vi "Polar Plot - Initialize Polar.vi"(6 "polar attributes":T2 {"minimum" format="%0.2f"; "maximum" format="%0.2f"}, 7 "[user-specified font]":T4, 11 "rect":T5={"left"=0, "top"=0, "right"=324, "bottom"=234}) -> (2 "grid measurements":T1 {"end angle" format="%0.2f"; "start angle" format="%0.2f"; "scale factors"."b" format="%0.2f"; "scale factors"."a" format="%0.2f"}, 3 "scale specs":cluster{"coordinate":i16, "label":string}[](array[cluster])=[{"coordinate"=7, "label"="1"}, {"coordinate"=23, "label"="2"}])   [LabVIEW 2020]
panel:
  in  "look up table":cluster{dbl, dbl}[](array[cluster])=[{0.0, 90.0}, {270.0, 360.0}, {180.0, 270.0}, {90.0, 180.0}, {0.0, 180.0}, {180.0, 360.0}, {270.0, 450.0}, {90.0, 270.0}, {0.0, 360.0}] {"?" format="%0.2f"; "?" format="%0.2f"}
  in  "desired font(Application)":T3(ring)=enum."Application Font"
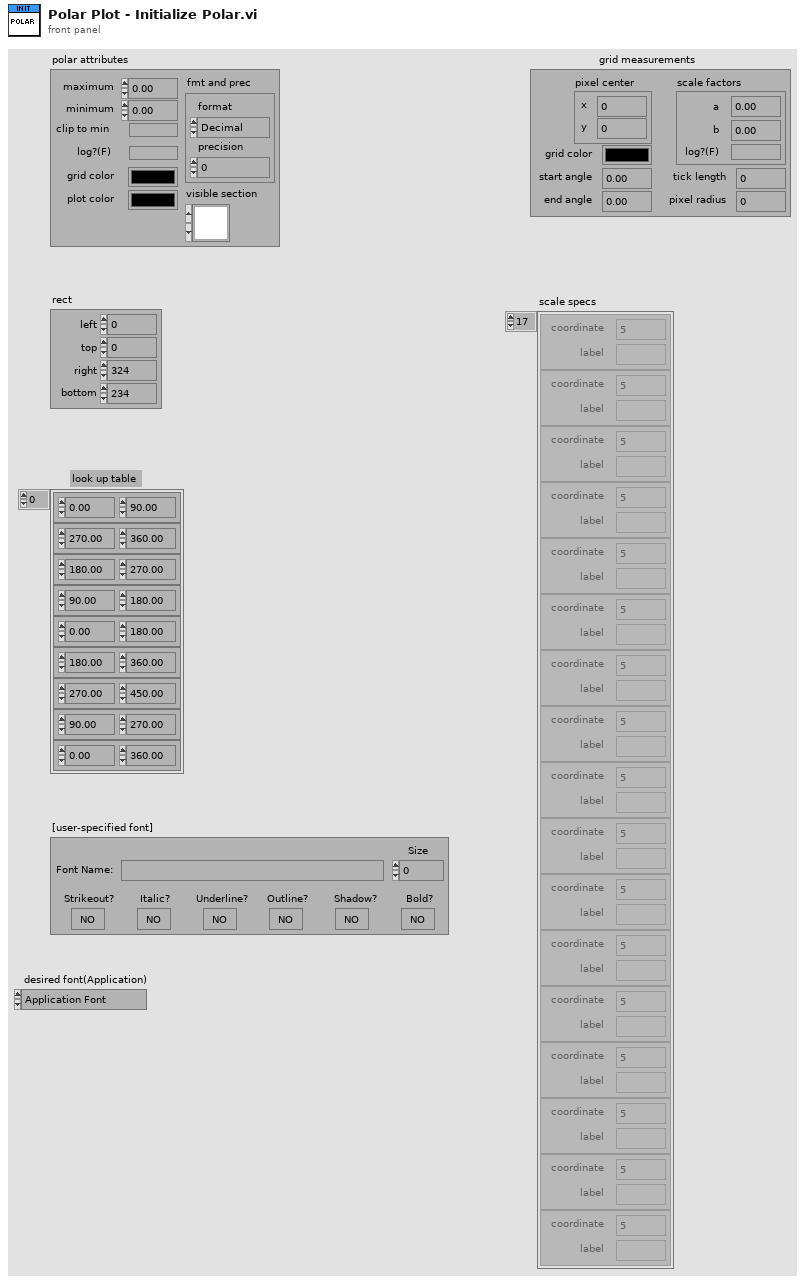
[diagram p1: front panel]
types:
  T1 = cluster{"pixel center":cluster{"x":i16, "y":i16}, "scale factors":cluster{"a":dbl, "b":dbl, "log?(F)":bool}, "grid color":u32, "start angle":dbl, "end angle":dbl, "tick length":i16, "pixel radius":i32}
  T2 = cluster{"maximum":dbl, "minimum":dbl, "clip to min":bool, "log?(F)":bool, "grid color":u32, "plot color":u32, "fmt and prec":cluster{"format":enum8{"Decimal", "Scientific", "Engineering", "Binary", "Octal", "Hex"}, "precision":u8}, "visible section":u16}
  T3 = enum16{"User-specified Font", "Application Font", "System Font", "Dialog Font"}
  T4 = cluster{"Font Name:":string, "Size":i16, "Strikeout?":bool, "Italic?":bool, "Underline?":bool, "Outline?":bool, "Shadow?":bool, "Bold?":bool}
  T5 = cluster{"left":i16, "top":i16, "right":i16, "bottom":i16}
  T6 = cluster{"Coordinate 1":i32, "maximum":dbl, "Coordinate 2":i32, "minimum":dbl, "log?(F)":bool, "fmt and prec":cluster{"format":enum8{"Decimal", "Scientific", "Engineering", "Binary", "Octal", "Hex"}, "precision":u8}}
  T7 = cluster{"format":enum8{"Decimal", "Scientific", "Engineering", "Binary", "Octal", "Hex"}, "precision":u8}
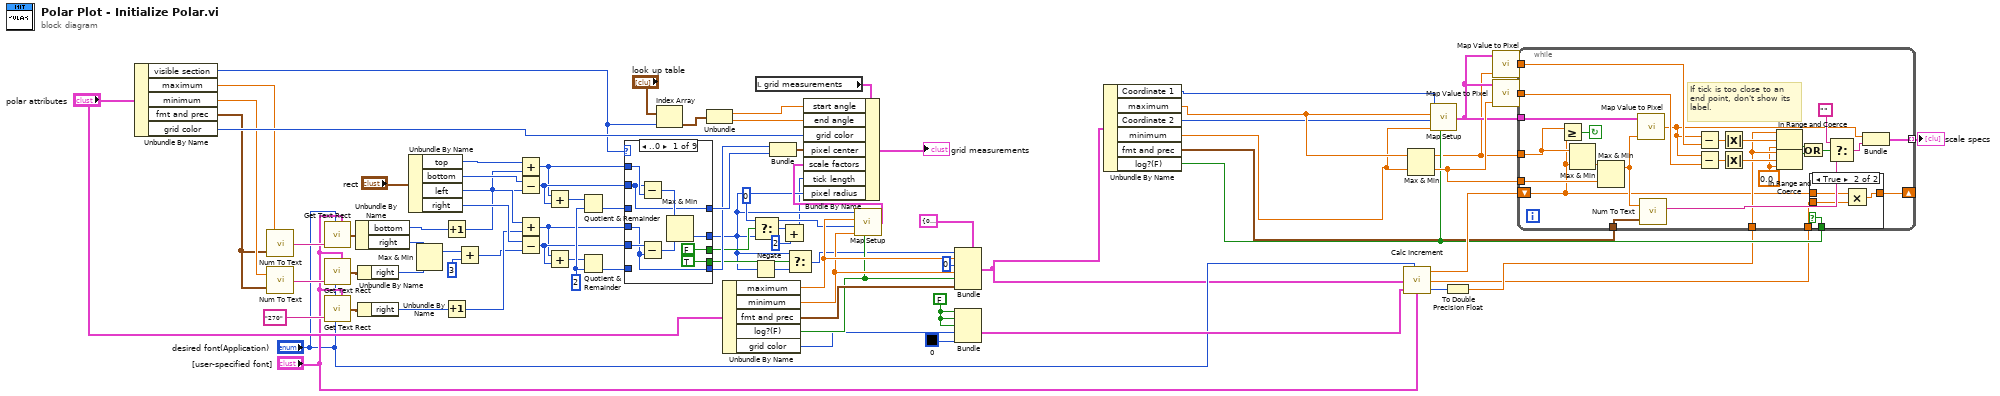
[diagram p0: block diagram]
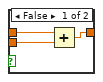
[diagram p2: hidden frame]
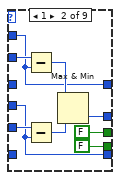
[diagram p3: hidden frame]
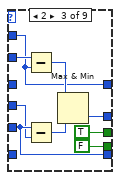
[diagram p4: hidden frame]
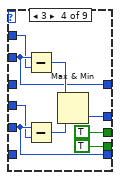
[diagram p5: hidden frame]
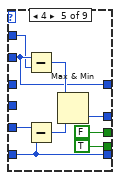
[diagram p6: hidden frame]
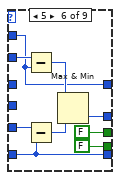
[diagram p7: hidden frame]
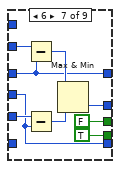
[diagram p8: hidden frame]
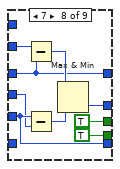
[diagram p9: hidden frame]
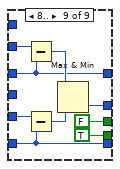
[diagram p10: hidden frame]
diagram:
  w31 = 0
  w67 = FALSE
  w78 = 2
  n1 = Unbundle By Name("polar attributes") -> ("visible section"=w25:u16, "maximum"=w54:dbl, "minimum"=w60:dbl, "fmt and prec"=w53:T7, "grid color"=w68:u32)
  n2 = call <vilib>:"Num To Text.vi"("fmt and prec"=w53, "number"=w54) -> ("numeric string"=w52:string)
  n3 = call <vilib>:"Num To Text.vi"("fmt and prec"=w53, "number"=w60) -> ("numeric string"=w75:string)
  n4 = call <vilib>:"Get Text Rect.vi"("desired font(Application)"="desired font(Application)", "text"=w52, "[user-specified font]"="[user-specified font]") -> ("rect"=w51:T5)  [unwired: 6 in]
  n5 = call <vilib>:"Get Text Rect.vi"("desired font(Application)"="desired font(Application)", "text"=w75, "[user-specified font]"="[user-specified font]") -> ("rect"=w74:T5)  [unwired: 6 in]
  n6 = call <vilib>:"Get Text Rect.vi"("desired font(Application)"="desired font(Application)", "text"="270", "[user-specified font]"="[user-specified font]") -> ("rect"=w73:T5)  [unwired: 6 in]
  n7 = Unbundle By Name(w51) -> ("bottom"=w48:i16, "right"=w50:i16)
  n8 = Unbundle By Name(w74) -> ("right"=w49:i16)
  n9 = Unbundle By Name(w73) -> ("right"=w46:i16)
  n10 = Unbundle By Name("rect") -> ("top"=w82:i16, "bottom"=w81:i16, "left"=w80:i16, "right"=w79:i16)
  n11 = Max & Min(x=w50, y=w49) -> (max(x,y)=w28:i16)  [unwired: 1 out]
  n12 = Increment(x=w48) -> (x+1=w47:i16)
  n13 = Increment(x=w46) -> (x+1=w45:i16)
  n14 = Add(x=w28, y=3) -> (x+y=w29:i32)
  n15 = Add(x=w82, y=w47) -> (x+y=w39:i16)
  n16 = Subtract(x=w81, y=w47) -> (x-y=w40:i16)
  n17 = Add(x=w80, y=w45) -> (x+y=w41:i16)
  n18 = Subtract(x=w79, y=w29) -> (x-y=w42:i32)
  n19 = Add(x=w39, y=w40) -> (x+y=w77:i16)
  n20 = Add(x=w41, y=w42) -> (x+y=w76:i32)
  n21 = Quotient & Remainder(x=w77, y=w78) -> (floor(x/y)=w38:i32)  [unwired: 1 out]
  n22 = Quotient & Remainder(x=w76, y=w78) -> (floor(x/y)=w43:i32)  [unwired: 1 out]
  n23 = case shown="..0" w25 {
    tunnel: w43 -> [_ _ _ _ w124 w131 _ _ w158]
    tunnel: w42 -> [w90 w98 w105 w115 w126 w134 w141 w150 w161]
    tunnel: w41 -> [w88 w96 w104 w113 _ _ w140 w149 _]
    tunnel: w38 -> [_ _ _ _ _ _ w142 w151 w159]
    tunnel: w40 -> [w86 w99 w108 w116 w123 w135 w144 w153 w162]
    tunnel: w39 -> [w87 w95 w106 w114 w122 w132 _ _ _]
    tunnel: [w89 w97 w107 w117 w125 w133 w143 w152 w160] -> w30
    tunnel: [w86 w95 w106 w116 w123 w132 w142 w151 w159] -> w37
    tunnel: [w88 w96 w105 w115 w124 w131 w140 w150 w158] -> w36
    tunnel: [TRUE FALSE FALSE TRUE TRUE FALSE TRUE TRUE TRUE] -> w35
    tunnel: [FALSE FALSE TRUE TRUE FALSE FALSE FALSE TRUE FALSE] -> w32
    frame ..0 {
      n24 = Subtract(x=w86, y=w87) -> (x-y=w91:i16)
      n25 = Subtract(x=w90, y=w88) -> (x-y=w92:i32)
      n26 = Max & Min(x=w91, y=w92) -> (min(x,y)=w89:i32)  [unwired: 1 out]
    }
    frame 1 {
      n27 = Subtract(x=w99, y=w95) -> (x-y=w100:i16)
      n28 = Subtract(x=w98, y=w96) -> (x-y=w101:i32)
      n29 = Max & Min(x=w100, y=w101) -> (min(x,y)=w97:i32)  [unwired: 1 out]
    }
    frame 2 {
      n30 = Subtract(x=w108, y=w106) -> (x-y=w109:i16)
      n31 = Subtract(x=w105, y=w104) -> (x-y=w110:i32)
      n32 = Max & Min(x=w109, y=w110) -> (min(x,y)=w107:i32)  [unwired: 1 out]
    }
    frame 3 {
      n33 = Subtract(x=w116, y=w114) -> (x-y=w118:i16)
      n34 = Subtract(x=w115, y=w113) -> (x-y=w119:i32)
      n35 = Max & Min(x=w118, y=w119) -> (min(x,y)=w117:i32)  [unwired: 1 out]
    }
    frame 4 {
      n36 = Subtract(x=w123, y=w122) -> (x-y=w127:i16)
      n37 = Subtract(x=w126, y=w124) -> (x-y=w128:i32)
      n38 = Max & Min(x=w127, y=w128) -> (min(x,y)=w125:i32)  [unwired: 1 out]
    }
    frame 5 {
      n39 = Subtract(x=w135, y=w132) -> (x-y=w136:i16)
      n40 = Subtract(x=w134, y=w131) -> (x-y=w137:i32)
      n41 = Max & Min(x=w136, y=w137) -> (min(x,y)=w133:i32)  [unwired: 1 out]
    }
    frame 6 {
      n42 = Subtract(x=w144, y=w142) -> (x-y=w145:i32)
      n43 = Subtract(x=w141, y=w140) -> (x-y=w146:i32)
      n44 = Max & Min(x=w145, y=w146) -> (min(x,y)=w143:i32)  [unwired: 1 out]
    }
    frame 7 {
      n45 = Subtract(x=w153, y=w151) -> (x-y=w154:i32)
      n46 = Subtract(x=w150, y=w149) -> (x-y=w155:i32)
      n47 = Max & Min(x=w154, y=w155) -> (min(x,y)=w152:i32)  [unwired: 1 out]
    }
    frame 8.. {
      n48 = Subtract(x=w162, y=w159) -> (x-y=w163:i32)
      n49 = Subtract(x=w161, y=w158) -> (x-y=w164:i32)
      n50 = Max & Min(x=w163, y=w164) -> (min(x,y)=w160:i32)  [unwired: 1 out]
    }
  }
  n51 = Index Array(array="look up table", index=w25) -> (element=w64:cluster{dbl, dbl})
  n52 = Unbundle(w64) -> (w62:dbl, w63:dbl)
  n53 = Unbundle By Name("polar attributes") -> ("maximum"=w57:dbl, "minimum"=w56:dbl, "fmt and prec"=w61:T7, "log?(F)"=w55:bool, "grid color"=w24:u32)
  n54 = Negate(x=w30) -> (-x=w33:i32)
  n55 = Select(t=w31, s=w32, f=w30) -> (s? t:f=w27:i32)
  n56 = local read "grid measurements"() -> (w69:T1)
  n57 = Bundle(w36, w37) -> (w59:cluster{i32, i32})  [unwired: 1 in]
  n58 = Add(x=w27, y=2) -> (x+y=w22:i32)
  n59 = Select(t=w30, s=w35, f=w33) -> (s? t:f=w34:i32)
  n60 = call <vilib>:"Map Setup.vi"("coordinate 1"=w30, "value 1"=w57, "coordinate 2"=w31, "value 2"=w56, "log?(F)"=w55) -> ("scale factors"=w58:cluster{"a":dbl, "b":dbl, "log?(F)":bool})
  n61 = Bundle By Name(cluster=w69, "start angle"=w62, "end angle"=w63, "grid color"=w68, "pixel center"=w59, "scale factors"=w58, "tick length"=w22, "pixel radius"=w30) -> (→"grid measurements":T1)
  n62 = Bundle(cluster=T6 {"Coordinate 1"=0, "maximum"=0.0, "Coordinate 2"=0, "minimum"=0.0, "log?(F)"=FALSE, "fmt and prec"={"format"=enum."Decimal", "precision"=0}}, "Coordinate 1"=w34, "maximum"=w57, "Coordinate 2"=0, "minimum"=w56, "log?(F)"=w55, "fmt and prec"=w61) -> (w5:T6)
  n63 = Bundle(w67, w67, w67, "grid color"=w24, u32 0) -> (w14:cluster{bool, bool, bool, "grid color":u32, u32})  [unwired: 1 in]
  n64 = Unbundle By Name(w5) -> ("Coordinate 1"=w12:i32, "maximum"=w11:dbl, "Coordinate 2"=w10:i32, "minimum"=w9:dbl, "fmt and prec"=w8:T7, "log?(F)"=w7:bool)
  n65 = call <vilib>:"Calc Increment.vi"("desired font(Application)"="desired font(Application)", "scale definition"=w5, "scale attributes"=w14, "[user-specified font]"="[user-specified font]") -> ("start"=w17:dbl, "increment"=w1:dbl, "text size"=w3:i16)  [unwired: 3 in]
  n66 = Max & Min(x=w11, y=w9) -> (max(x,y)=w4:dbl, min(x,y)=w21:dbl)
  n67 = call <vilib>:"Map Setup.vi"("coordinate 1"=w12, "value 1"=w11, "coordinate 2"=w10, "value 2"=w9, "log?(F)"=w7) -> ("scale factors"=w20:cluster{"a":dbl, "b":dbl, "log?(F)":bool})
  n68 = To Double Precision Float(number=w3) -> (double precision float=w2:dbl)
  n69 = call <vilib>:"Map Value to Pixel.vi"("x"=w4, "scale factors"=w20) -> ("pixel"=w19:dbl)  [unwired: 1 in]
  n70 = call <vilib>:"Map Value to Pixel.vi"("x"=w21, "scale factors"=w20) -> ("pixel"=w18:dbl)  [unwired: 1 in]
  n71 = while {
    tunnel: w7 -> [w165]
    tunnel: w18 -> [w175]
    tunnel: w19 -> [w183]
    tunnel: w2 -> [w174]
    tunnel: w8 -> [w186]
    tunnel: [w190] -> w16 mode=indexing
    tunnel: w1 -> [w168]
    tunnel: w20 -> [w185]
    tunnel: w21 -> [w188]
    tunnel: w4 -> [w187]
    shift-left: w17 -> [w167]
    shift-right: [w166] -> _
    stop <- w189 continue-if-true
    w173 = 0.0
    # "If tick is too close to an\nend point, don't show its\nlabel."
    n72 = Greater Or Equal?(x=w187, y=w167) -> (x >= y?=w189:bool)
    n73 = Max & Min(x=w187, y=w167) -> (min(x,y)=w191:dbl)  [unwired: 1 out]
    n74 = Max & Min(x=w191, y=w188) -> (max(x,y)=w184:dbl)  [unwired: 1 out]
    n75 = call <vilib>:"Map Value to Pixel.vi"("x"=w184, "scale factors"=w185) -> ("pixel"=w169:dbl)  [unwired: 1 in]
    n76 = call <vilib>:"Num To Text.vi"("fmt and prec"=w186, "number"=w184) -> ("numeric string"=w179:string)
    n77 = Subtract(x=w169, y=w183) -> (x-y=w182:dbl)
    n78 = Subtract(x=w169, y=w175) -> (x-y=w176:dbl)
    n79 = Absolute Value(x=w182) -> (abs(x)=w181:dbl)
    n80 = Absolute Value(x=w176) -> (abs(x)=w177:dbl)
    n81 = In Range and Coerce(upper limit=w174, x=w181, lower limit=w173) -> (In Range?=w171:bool)  [unwired: 1 out]
    n82 = In Range and Coerce(upper limit=w174, x=w177, lower limit=w173) -> (In Range?=w170:bool)  [unwired: 1 out]
    n83 = Or(x=w171, y=w170) -> (x .or. y?=w172:bool)
    n84 = case shown="True" w165 {
      tunnel: w168 -> [w193 w197]
      tunnel: w167 -> [w192 w196]
      tunnel: [w194 w195] -> w166
      frame False {
        n85 = Add(x=w192, y=w193) -> (x+y=w194:dbl)
      }
      frame True {
        n86 = Multiply(x=w196, y=w197) -> (x*y=w195:dbl)
      }
    }
    n87 = Select(t="", s=w172, f=w179) -> (s? t:f=w178:string)
    n88 = Bundle("pixel"=w169, "numeric string"=w178) -> (w190:cluster{"pixel":dbl, "numeric string":string})  [unwired: 1 in]
  }
  "scale specs" <- w16
